vi "DO增加一条自动检测记录.vi"(8 "测试结果":string, 10 "测试内容":string) -> ()   [LabVIEW 2010]
uses:
  全局量/自动测试结果.vi
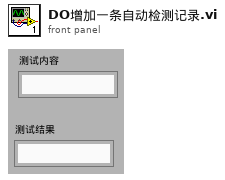
[diagram p1: front panel]
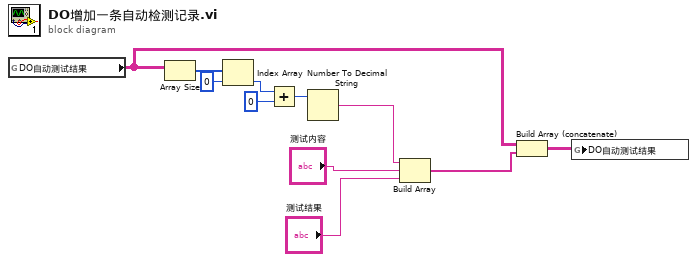
[diagram p0: block diagram]
diagram:
  n1 = global read "自动测试结果.vi" "DO自动测试结果"() -> (w3:string[][])
  n2 = Array Size(array=w3) -> (size(s)=w11:i32[])
  n3 = Index Array(array=w11, index=0 ("索引")) -> (element=w9:i32)
  n4 = Add(x=w9, y=0) -> (x+y=w7:i32)
  n5 = Number To Decimal String(number=w7) -> (decimal integer string=w6:string)  [unwired: 1 in]
  n6 = Build Array(w6, "测试内容", "测试结果") -> (w2:string[])
  n7 = Build Array (concatenate)(w3, w2) -> (w1:string[][])
  n8 = global write "自动测试结果.vi" "DO自动测试结果"(w1) -> ()
